vi "Distort Image (ARGB).vi"(5 "Border Type (Default: Constant)":T2, 6 "Use Fixed Point Remapping (Default: False)":bool, 7 "ARGB Colour (Default: Black)":T1={"Alpha"=255, "RGB"=0}, 8 "error in (no error)":errorcluster, 9 "ARGB Image Destination in":T3, 10 "ARGB Image Source in":T3, 11 "Image Distorter in":refnum<class "Image Distorter.lvclass">) -> (0 "error out":errorcluster, 2 "ARGB Image Destination":T3, 3 "Image Distorter":refnum<class "Image Distorter.lvclass">)   [LabVIEW 2020, in "image.lvlib" / "Image Distorter.lvclass"]
doc: "Apply distortion to the Source Image."
uses:
  Image Distorter.lvclass
  ARGB Image.ctl
  Border Type.ctl
  ARGB Colour.ctl
  Image Distorter.lvclass/Image Distorter.ctl
  ccc224f2-fea8-4097-85c8-c2b3fe04188f.vi
  <vilib>/Utility/error.llb/Error Cluster From Error Code.vi
  image.lvlib
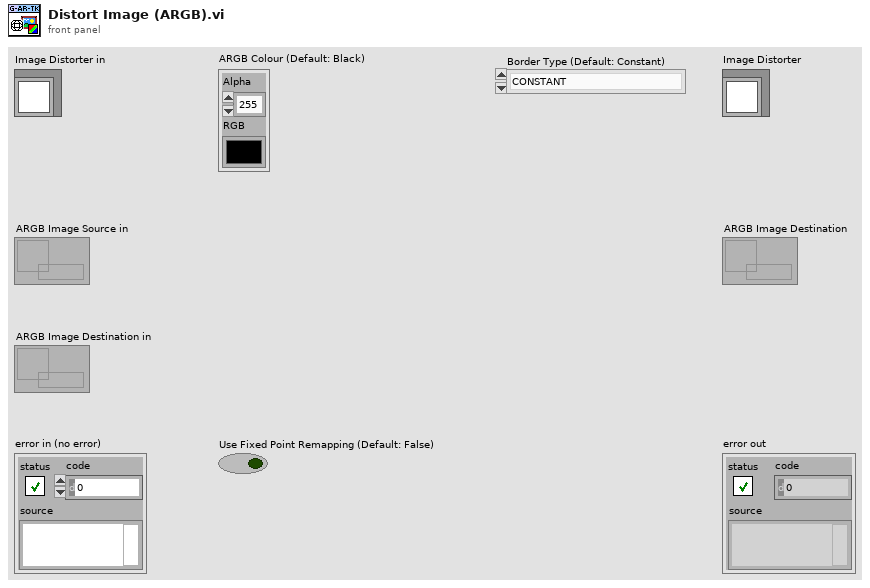
[diagram p1: front panel]
types:
  T1 = typedef "image.lvlib/ARGB Colour.ctl" = cluster{"Alpha":u8, "RGB":u32}
  T2 = typedef "image.lvlib/Border Type.ctl" = enum8{"CONSTANT", "REPLICATE", "REFLECT", "WRAP", "TRANSPARENT", "DEFAULT", "ISOLATED"}
  T3 = typedef "image.lvlib/ARGB Image.ctl" = refnum<data-value>
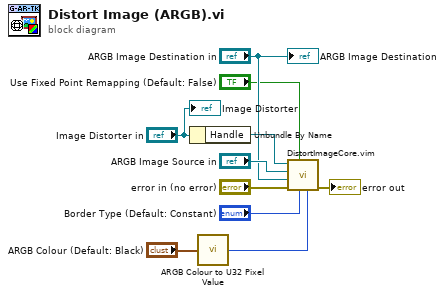
[diagram p0: block diagram]
diagram:
  n1 = Unbundle By Name("Image Distorter in") -> ("Handle"=w9:refnum<data-value>)
  n2 = call "ARGB Colour to U32 Pixel Value.vi"("ARGB Colour"="ARGB Colour (Default: Black)") -> ("U32 Colour"=w1:u32)
  n3 = call "DistortImageCore.vim"("Colour"=w1, "Border Type"="Border Type (Default: Constant)", "Use Fixed Point remapping"="Use Fixed Point Remapping (Default: False)", "error in (no error)"="error in (no error)", "Destination Image"="ARGB Image Destination in", "Source Image"="ARGB Image Source in", "Handle"=w9) -> ("error out"=→"error out":errorcluster)  [unwired: 4 in]
  "Image Distorter" <- "Image Distorter in"
  "ARGB Image Destination" <- "ARGB Image Destination in"
